vi "Manage Robot Shape.vi"(4 "Lighter":bool, 6 "Coords":cluster{"x":dbl, "y":dbl}, 7 "Drawing Options":T1, 8 "Operation":enum16{"Draw", "Pt Test"}(ring), 9 "new picture in":picture, 10 "Robot Position (ft)":cluster{"x":dbl, "y":dbl, "th":dbl}, 11 "Pict Ref":refnum<vi>) -> (0 "Pt Test Results":enum16{"Miss", "Rect Hit", "Arrow Hit"}(ring), 1 "new picture out":picture, 2 "Boundary Poly":cluster{dbl, dbl}[](array[cluster]))   [LabVIEW 2018]
uses:
  <vilib>/Analysis/geometry.llb/Point in Polygon Position.ctl
  <vilib>/Analysis/geometry.llb/Point in Polygon (Scalar).vi
  <vilib>/Analysis/NI_AAL_Geometry.lvlib
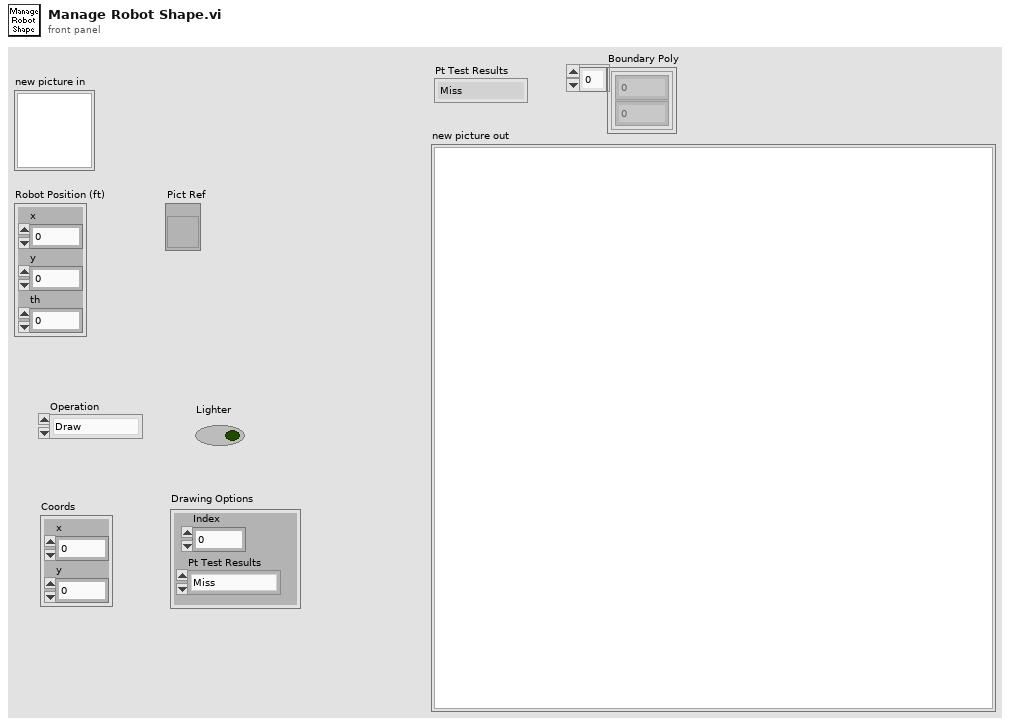
[diagram p1: front panel]
types:
  T1 = cluster{"Index":u32, "Pt Test Results":enum16{"Miss", "Rect Hit", "Arrow Hit"}}
  T2 = typedef "LVPositionTypeDef.ctl" = cluster{"Left":i32, "Top":i32}
  T3 = typedef "LVBoundsTypeDef.ctl" = cluster{"Width":u32, "Height":u32}
  T4 = cluster{"Width":u16, "Style":enum32{"Solid", "Dash", "Dot", "DashDot", "DashDotDot"}}
  T5 = typedef "NI_AAL_Geometry.lvlib/Point in Polygon Position.ctl" = u16
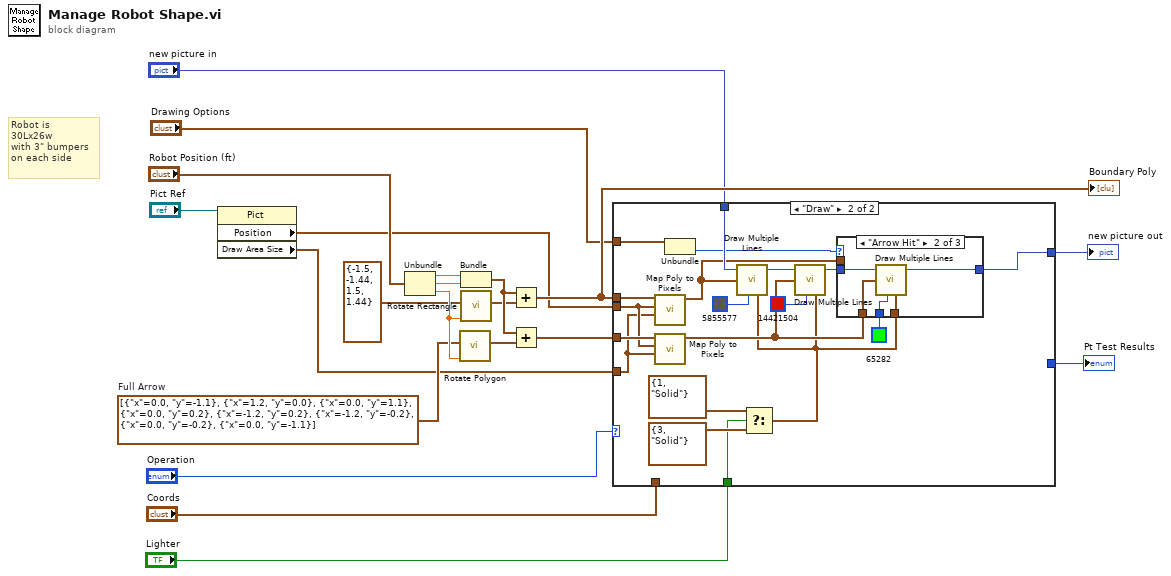
[diagram p0: block diagram]
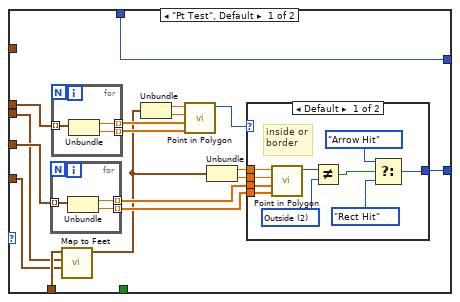
[diagram p2: hidden frame]
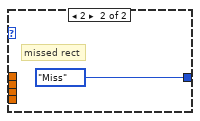
[diagram p3: hidden frame]
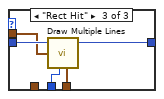
[diagram p5: hidden frame]
diagram:
  w10 = cluster{"x":dbl, "y":dbl}[] [{"x"=0.0, "y"=-1.1}, {"x"=1.2, "y"=0.0}, {"x"=0.0, "y"=1.1}, {"x"=0.0, "y"=0.2}, {"x"=-1.2, "y"=0.2}, {"x"=-1.2, "y"=-0.2}, {"x"=0.0, "y"=-0.2}, {"x"=0.0, "y"=-1.1}]  # Full Arrow
  # "Robot is\n30Lx26w\nwith 3\" bumpers\non each side"
  n1 = property on="Property Node" class="Pict"(reference="Pict Ref") -> ("Position"=w8:T2, "Draw Area Size"=w7:T3)  [unwired: 1 in, 2 out]
  n2 = Unbundle("Robot Position (ft)") -> ("x"=w12:dbl, "y"=w13:dbl, "th"=w15:dbl)
  n3 = call "Rotate Polygon.vi"("Angle"=w15, "polygon 2"=w10) -> ("polygon"=w19:cluster{dbl, dbl}[])  [unwired: 9 in]
  n4 = Bundle("x"=w12, "y"=w13) -> (w21:cluster{"x":dbl, "y":dbl})  [unwired: 1 in]
  n5 = call "Rotate Rectangle.vi"("Angle"=w15, "Rectangle"=cluster{"x":dbl, "y":dbl, "x":dbl, "y":dbl} {"x"=-1.5, "y"=-1.44, "x"=1.5, "y"=1.44} ("output cluster")) -> ("polygon"=w18:cluster{dbl, dbl}[])  [unwired: 9 in]
  n6 = Add(x=w21, y=w18) -> (x+y=w17:cluster{dbl, dbl}[])
  "Boundary Poly" <- w17
  n7 = Add(x=w21, y=w19) -> (x+y=w20:cluster{dbl, dbl}[])
  n8 = case shown="\"Draw\"" "Operation" {
    tunnel: w20 -> [w32 w74]
    tunnel: w17 -> [w34 w73]
    tunnel: [w33 w66] -> w16
    tunnel: "new picture in" -> [w33 w70]
    tunnel: w8 -> [w22 w69]
    tunnel: w7 -> [w23 w68]
    tunnel: "Coords" -> [w24 _]
    tunnel: [w26 _] -> w3
    tunnel: "Drawing Options" -> [_ w63]
    tunnel: "Lighter" -> [_ w58]
    frame "Pt Test", Default {
      n9 = for {
        tunnel: w32 -> [w52] mode=indexing
        tunnel: [w51] -> w28 mode=indexing
        tunnel: [w50] -> w27 mode=indexing
        n10 = Unbundle(w52) -> (w51:dbl, w50:dbl)
      }
      n11 = for {
        tunnel: w34 -> [w55] mode=indexing
        tunnel: [w54] -> w37 mode=indexing
        tunnel: [w53] -> w38 mode=indexing
        n12 = Unbundle(w55) -> (w54:dbl, w53:dbl)
      }
      n13 = call "Map to Feet.vi"("Draw Area Size"=w23, "Position"=w22, "Coords (px)"=w24) -> ("Point (ft)"=w25:cluster{dbl, dbl})  [unwired: 8 in]
      n14 = Unbundle(w25) -> (w36:dbl, w35:dbl)
      n15 = call-poly <vilib>:"Point in Polygon.vi"("Polygon Y"=w38, "Polygon X"=w37, "y"=w35, "x"=w36) -> ("position"=w31:T5)  [unwired: 6 in, 1 out]
      n16 = Unbundle(w25) -> (w30:dbl, w29:dbl)
      n17 = case shown="Default" w31 {
        tunnel: w30 -> [w48 _]
        tunnel: w29 -> [w47 _]
        tunnel: w28 -> [w46 _]
        tunnel: w27 -> [w45 _]
        tunnel: [w40 enum16{"Miss", "Rect Hit", "Arrow Hit"}."Miss" ("Pt Test Results")] -> w26
        frame Default {
          w44 = T5 2 items=["Inside", "On Boundary", "Outside"] ("position")
          # "inside or\nborder"
          n18 = call-poly <vilib>:"Point in Polygon.vi"("Polygon Y"=w45, "Polygon X"=w46, "y"=w47, "x"=w48) -> ("position"=w43:T5)  [unwired: 6 in, 1 out]
          n19 = Not Equal?(x=w43, y=w44) -> (x != y?=w39:bool)
          n20 = Select(t=enum16{"Miss", "Rect Hit", "Arrow Hit"}."Arrow Hit" ("Pt Test Results"), s=w39, f=enum16{"Miss", "Rect Hit", "Arrow Hit"}."Rect Hit" ("Pt Test Results")) -> (s? t:f=w40:enum16{"Miss", "Rect Hit", "Arrow Hit"})
        }
        frame 2 {
          # "missed rect"
        }
      }
    }
    frame "Draw" {
      n21 = call "Map Poly to Pixels.vi"("Draw Area Size"=w68, "Position"=w69, "Coords"=w73) -> ("Coords"=w62:cluster{"Horizontal":dbl, "Vertical":dbl}[])  [unwired: 8 in]
      n22 = call "Map Poly to Pixels.vi"("Draw Area Size"=w68, "Position"=w69, "Coords"=w74) -> ("Coords"=w65:cluster{"Horizontal":dbl, "Vertical":dbl}[])  [unwired: 8 in]
      n23 = Unbundle(w63) -> ("Pt Test Results"=w61:enum16{"Miss", "Rect Hit", "Arrow Hit"})  [unwired: 1 out]
      n24 = Select(t=T4 {"Width"=1, "Style"=enum."Solid"} ("pen"), s=w58, f=T4 {"Width"=3, "Style"=enum."Solid"} ("pen")) -> (s? t:f=w57:T4)
      n25 = call <vilib>:"Draw Multiple Lines.vi"("picture"=w70, "line endpoints"=w62, "color(black)"=u32 5855577, "pen"=w57) -> ("new picture"=w71:picture)  [unwired: 5 in]
      n26 = call <vilib>:"Draw Multiple Lines.vi"("picture"=w71, "line endpoints"=w65, "color(black)"=u32 14421504, "pen"=w57) -> ("new picture"=w67:picture)  [unwired: 5 in]
      n27 = case shown="\"Arrow Hit\"" w61 {
        tunnel: w67 -> [w75 w80 w85]
        tunnel: [w75 w79 w84] -> w66
        tunnel: w65 -> [_ w78 _]
        tunnel: u32 65282 ("color(black)") -> [_ w77 w83]
        tunnel: w62 -> [_ _ w82]
        tunnel: w57 -> [_ w76 w81]
        frame Default {
        }
        frame "Arrow Hit" {
          n28 = call <vilib>:"Draw Multiple Lines.vi"("picture"=w80, "line endpoints"=w78, "color(black)"=w77, "pen"=w76) -> ("new picture"=w79:picture)  [unwired: 5 in]
        }
        frame "Rect Hit" {
          n29 = call <vilib>:"Draw Multiple Lines.vi"("picture"=w85, "line endpoints"=w82, "color(black)"=w83, "pen"=w81) -> ("new picture"=w84:picture)  [unwired: 5 in]
        }
      }
    }
  }
  "new picture out" <- w16
  "Pt Test Results" <- w3
